vi "Test.vi"() -> ()   [LabVIEW 2017]
doc: "This VI is called when test mode begins, and will automatically be terminated when it ends. You can add manual or automatic tests and invoke them from the dashboard."
uses:
  <vilib>/Rock Robotics/WPI/Utilities/WPI_GetSetVariantRefNum.vi
panel:
  out "Elapsed Time (s) 2":dbl caption="Elapsed Time (s)"
  out "Elapsed Time (s)":dbl
  out "Distance 24":dbl
  out "Distance 23":dbl
  out "Distance 22":dbl
  out "Distance 21":dbl
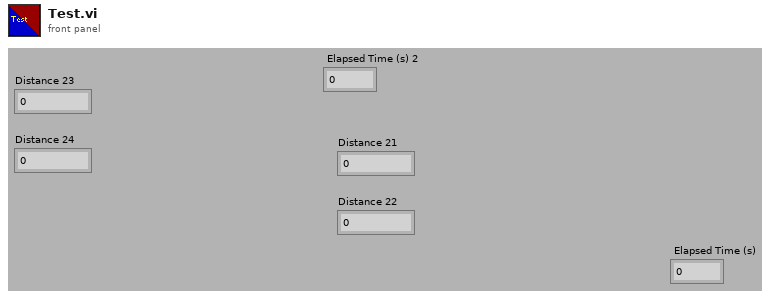
[diagram p1: front panel]
types:
  T1 = typedef "WPI_EncoderDevRef.ctl" = cluster{"DevStatus":errorcluster, "EncoderIndex":T2, "CounterIndex":T3, "DistancePerCount":dbl, "Decoding Type":T4}
  T2 = typedef "FPGA_EncoderIdx.ctl" = enum8{"Enc 0", "Enc 1", "Enc 2", "Enc 3", "Enc 4", "Enc 5", "Enc 6", "Enc 7", "Invalid"}
  T3 = typedef "FPGA_CounterCtrSystemIndex.ctl" = enum8{"Ctr 0", "Ctr 1", "Ctr 2", "Ctr 3", "Ctr 4", "Ctr 5", "Ctr 6", "Ctr 7", "Invalid"}
  T4 = typedef "WPI_EncoderType.ctl" = enum16{"1x", "2x", "4x"}
  T5 = typedef "WPI_RobotDriveDevRef.ctl" = cluster{"DevStatus":errorcluster, "Motors[]":T6[], "Square Inputs":bool, "Max Output":dbl}
  T6 = typedef "WPI_MotorControlDeviceRef.ctl" = cluster{"DeviceStatus":errorcluster, "Type":T7, "PWM":cluster{"PWM Channel":T8, "DeadBand":T9}, "CAN":cluster{"Device Number":u8, "SetOutput VI Ref":variant, "GetOutput VI Ref":variant, "Enable VI Ref":variant, "Disable VI Ref":variant, "Data":variant}, "Invert":bool, "DIO PWM":cluster{"PWM \"Enable\" Channel":T8, "DIOChannel":T10, "PWM Rate":dbl}}
  T7 = typedef "WPI_MotorControlType.ctl" = enum16{"PWM", "CAN", "DIO PWM"}
  T8 = typedef "FPGA_DIOPWMChannel.ctl" = enum8{"PWM 0", "PWM 1", "PWM 2", "PWM 3", "PWM 4", "PWM 5", "PWM 6", "PWM 7", "PWM 8", "PWM 9", "PWM MXP 0", "PWM MXP 1", "PWM MXP 2", "PWM MXP 3", "PWM MXP 4", "PWM MXP 5", "PWM MXP 6", "PWM MXP 7", "PWM MXP 8", "PWM MXP 9", "Invalid"}
  T9 = typedef "WPI_PWMDeadband.ctl" = cluster{"Name":string, "maxPositivePwm":i32, "minPositivePwm":i32, "centerPwm":i32, "maxNegativePwm":i32, "minNegativePwm":i32, "angularRange":u16}
  T10 = typedef "FPGA_DIOChannel.ctl" = enum8{"DIO 0", "DIO 1", "DIO 2", "DIO 3", "DIO 4", "DIO 5", "DIO 6", "DIO 7", "DIO 8", "DIO 9", "DIO MXP 0", "DIO MXP 1", "DIO MXP 2", "DIO MXP 3", "DIO MXP 4", "DIO MXP 5", "DIO MXP 6", "DIO MXP 7", "DIO MXP 8", "DIO MXP 9", "DIO MXP 10", "DIO MXP 11", "DIO MXP 12", "DIO MXP 13", "DIO MXP 14", "DIO MXP 15", "SPI Port CS1", "SPI Port CS2", "SPI Port CS3", "SPI Port MISO", "SPI Port MOSI", "Invalid"}
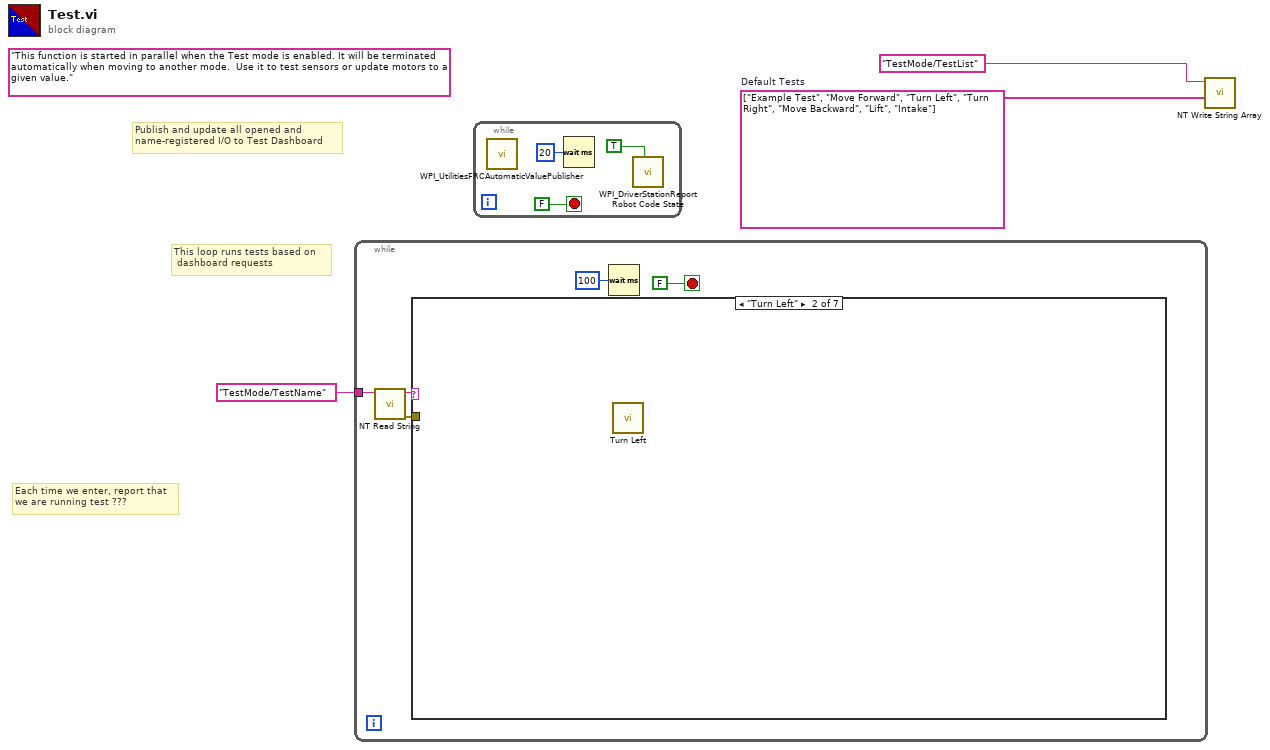
[diagram p0: block diagram]
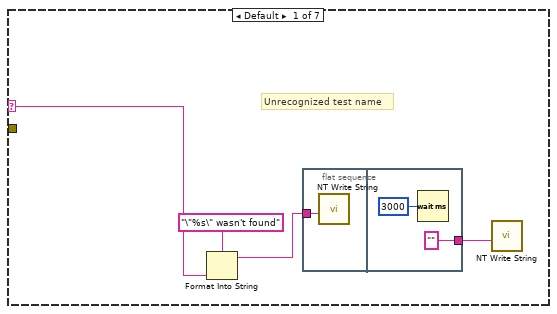
[diagram p2: hidden frame]
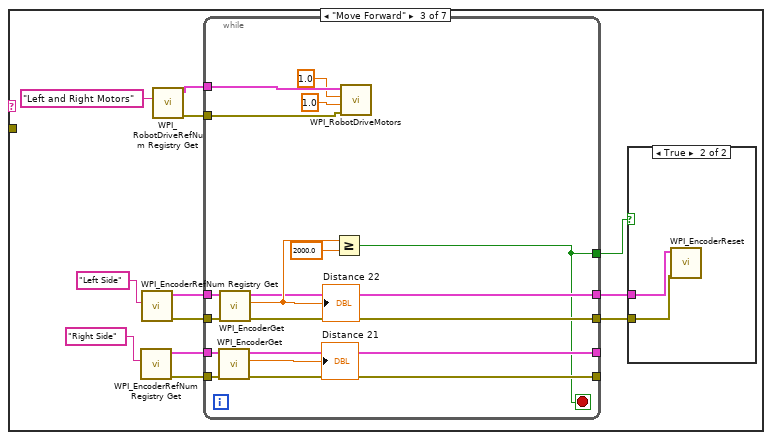
[diagram p3: hidden frame]
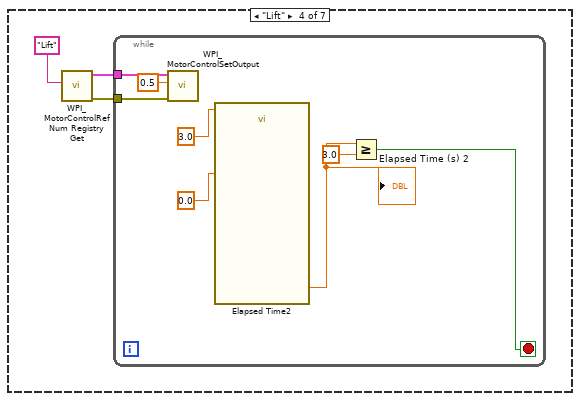
[diagram p5: hidden frame]
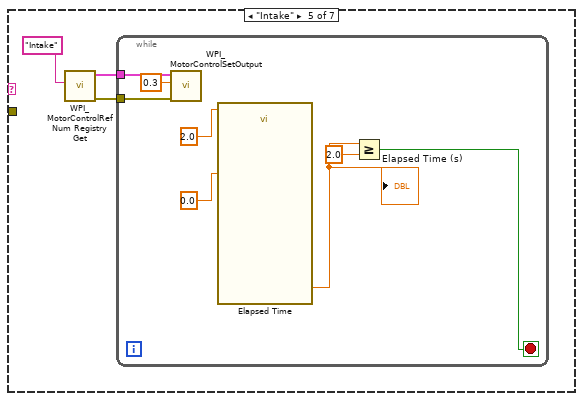
[diagram p6: hidden frame]
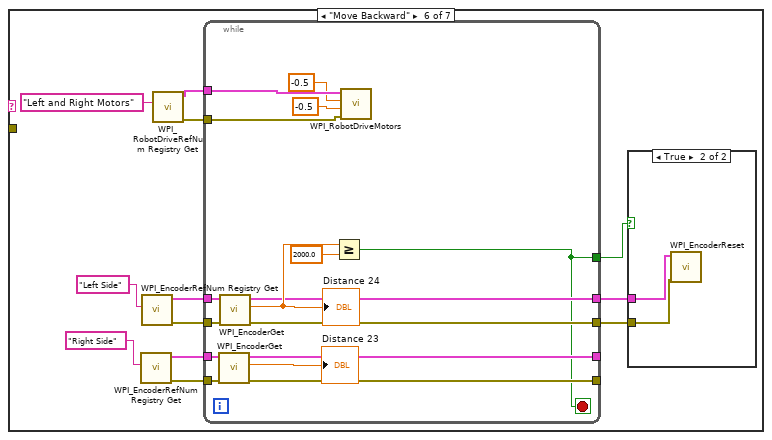
[diagram p7: hidden frame]
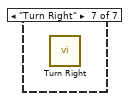
[diagram p9: hidden frame]
diagram:
  w2 = string[] ["Example Test", "Move Forward", "Turn Left", "Turn Right", "Move Backward", "Lift", "Intake"]  # Default Tests
  (unwired) "This function is started in parallel when the Test mode is enabled. It will be terminated automatically when moving to another mode.  Use it to test sensors or update motors to a given value."
  # "This loop runs tests based on \n dashboard requests"
  # "Publish and update all opened and\nname-registered I/O to Test Dashboard"
  # "Each time we enter, report that\nwe are running test ???"
  n1 = while {
    tunnel: "TestMode/TestName" ("Name") -> [w5]
    stop <- FALSE stop-if-true
    n2 = call <vilib>:"NT Read String.vi"("Name"=w5) -> ("error out"=w4:errorcluster, "String"=w6:string)  [unwired: 9 in]
    n3 = case shown="\"Turn Left\"" w6 {
      selector: w6 -> [w12 _ _ _ _ _ _]
      tunnel: w4 -> [_ _ _ _ _ _ _]
      frame Default {
        # "Unrecognized test name"
        n4 = Format Into String(format string="\"%s\" wasn't found" ("Name"), w12) -> (resulting string=w11:string)  [unwired: 2 in, 1 out]
        n5 = flat-sequence {
          tunnel: w11 -> [w13]
          tunnel: ["" ("Name")] -> w9
          frame #0 {
            n6 = call <vilib>:"NT Write String.vi"("String"=w13) -> ()  [unwired: 10 in, 1 out]
          }
          frame #1 {
            n7 = Wait (ms)(milliseconds to wait=u32 3000) -> ()  [unwired: 1 out]
          }
        }
        n8 = call <vilib>:"NT Write String.vi"("String"=w9) -> ()  [unwired: 10 in, 1 out]
      }
      frame "Turn Left" {
        n9 = call "Turn Left.vi"() -> ()  [unwired: 12 in]
      }
      frame "Move Forward" {
        n10 = call <vilib>:"WPI_EncoderRefNum Registry Get.vi"("refnum name"="Right Side") -> ("error out"=w25:errorcluster, "EncoderDevRef"=w24:T1)  [unwired: 9 in]
        n11 = call <vilib>:"WPI_EncoderRefNum Registry Get.vi"("refnum name"="Left Side") -> ("error out"=w26:errorcluster, "EncoderDevRef"=w27:T1)  [unwired: 9 in]
        n12 = call <vilib>:"WPI_RobotDriveRefNum Registry Get.vi"("refnum name"="Left and Right Motors") -> ("error out"=w19:errorcluster, "RobotDriveDevRef"=w20:T5)  [unwired: 9 in]
        n13 = while {
          tunnel: w27 -> [w45]
          tunnel: w26 -> [w44]
          tunnel: w24 -> [w41]
          tunnel: w25 -> [w42]
          tunnel: [w38] -> w22
          tunnel: [w37] -> w21
          tunnel: [w36] -> _
          tunnel: [w35] -> _
          tunnel: [w34] -> w23
          tunnel: w20 -> [w33]
          tunnel: w19 -> [w32]
          stop <- w34 stop-if-true
          n14 = call <vilib>:"WPI_EncoderGet.vi"("error in (no error)"=w42, "EncoderDevRef"=w41) -> ("error out"=w35:errorcluster, "Distance"=→"Distance 21":dbl, "EncoderDevRef"=w36:T1)  [unwired: 4 in, 3 out]
          n15 = call <vilib>:"WPI_EncoderGet.vi"("error in (no error)"=w44, "EncoderDevRef"=w45) -> ("error out"=w37:errorcluster, "Distance"=w40:dbl, "EncoderDevRef"=w38:T1)  [unwired: 4 in, 3 out]
          "Distance 22" <- w40
          n16 = Greater Or Equal?(x=w40, y=2000.0) -> (x >= y?=w34:bool)
          n17 = call <vilib>:"WPI_RobotDriveMotors.vi"("error in (no error)"=w32, "RightSpeed"=1.0, "LeftSpeed"=1.0, "RobotDriveDevRef"=w33) -> ()  [unwired: 5 in, 3 out]
        }
        n18 = case shown="True" w23 {
          tunnel: w22 -> [_ w29]
          tunnel: w21 -> [_ w28]
          frame False {
          }
          frame True {
            n19 = call <vilib>:"WPI_EncoderReset.vi"("error in (no error)"=w28, "EncoderDevRef"=w29) -> ()  [unwired: 8 in, 2 out]
          }
        }
      }
      frame "Lift" {
        n20 = call <vilib>:"WPI_MotorControlRefNum Registry Get.vi"("refnum name"="Lift") -> ("error out"=w47:errorcluster, "MotorControlDevRef"=w48:T6)  [unwired: 9 in]
        n21 = while {
          tunnel: w47 -> [w56]
          tunnel: w48 -> [w55]
          stop <- w49 stop-if-true
          n22 = call <vilib>:"WPI_MotorControlSetOutput.vi"("error in (no error)"=w56, "Output"=0.5, "MotorControlDevRef"=w55) -> ()  [unwired: 6 in, 3 out]
          n23 = call "Elapsed Time2"("Time Target (s)"=3.0, "Set Start Time (s)"=0.0) -> ("Elapsed Time (s)"=w53:dbl)  [unwired: 10 in, 7 out]
          "Elapsed Time (s) 2" <- w53
          n24 = Greater Or Equal?(x=w53, y=3.0) -> (x >= y?=w49:bool)
        }
      }
      frame "Intake" {
        n25 = call <vilib>:"WPI_MotorControlRefNum Registry Get.vi"("refnum name"="Intake") -> ("error out"=w58:errorcluster, "MotorControlDevRef"=w57:T6)  [unwired: 9 in]
        n26 = while {
          tunnel: w58 -> [w67]
          tunnel: w57 -> [w66]
          stop <- w60 stop-if-true
          n27 = call <vilib>:"WPI_MotorControlSetOutput.vi"("error in (no error)"=w67, "Output"=0.3, "MotorControlDevRef"=w66) -> ()  [unwired: 6 in, 3 out]
          n28 = call "Elapsed Time"("Time Target (s)"=2.0, "Set Start Time (s)"=0.0) -> ("Elapsed Time (s)"=w64:dbl)  [unwired: 10 in, 7 out]
          "Elapsed Time (s)" <- w64
          n29 = Greater Or Equal?(x=w64, y=2.0) -> (x >= y?=w60:bool)
        }
      }
      frame "Move Backward" {
        n30 = call <vilib>:"WPI_EncoderRefNum Registry Get.vi"("refnum name"="Right Side") -> ("error out"=w73:errorcluster, "EncoderDevRef"=w74:T1)  [unwired: 9 in]
        n31 = call <vilib>:"WPI_EncoderRefNum Registry Get.vi"("refnum name"="Left Side") -> ("error out"=w72:errorcluster, "EncoderDevRef"=w71:T1)  [unwired: 9 in]
        n32 = call <vilib>:"WPI_RobotDriveRefNum Registry Get.vi"("refnum name"="Left and Right Motors") -> ("error out"=w79:errorcluster, "RobotDriveDevRef"=w78:T5)  [unwired: 9 in]
        n33 = while {
          tunnel: w71 -> [w97]
          tunnel: w72 -> [w96]
          tunnel: w74 -> [w93]
          tunnel: w73 -> [w94]
          tunnel: [w90] -> w76
          tunnel: [w89] -> w77
          tunnel: [w88] -> _
          tunnel: [w87] -> _
          tunnel: [w86] -> w75
          tunnel: w78 -> [w85]
          tunnel: w79 -> [w84]
          stop <- w86 stop-if-true
          n34 = call <vilib>:"WPI_EncoderGet.vi"("error in (no error)"=w94, "EncoderDevRef"=w93) -> ("error out"=w87:errorcluster, "Distance"=→"Distance 23":dbl, "EncoderDevRef"=w88:T1)  [unwired: 4 in, 3 out]
          n35 = call <vilib>:"WPI_EncoderGet.vi"("error in (no error)"=w96, "EncoderDevRef"=w97) -> ("error out"=w89:errorcluster, "Distance"=w92:dbl, "EncoderDevRef"=w90:T1)  [unwired: 4 in, 3 out]
          "Distance 24" <- w92
          n36 = Greater Or Equal?(x=w92, y=2000.0) -> (x >= y?=w86:bool)
          n37 = call <vilib>:"WPI_RobotDriveMotors.vi"("error in (no error)"=w84, "RightSpeed"=-0.5, "LeftSpeed"=-0.5, "RobotDriveDevRef"=w85) -> ()  [unwired: 5 in, 3 out]
        }
        n38 = case shown="True" w75 {
          tunnel: w76 -> [_ w81]
          tunnel: w77 -> [_ w80]
          frame False {
          }
          frame True {
            n39 = call <vilib>:"WPI_EncoderReset.vi"("error in (no error)"=w80, "EncoderDevRef"=w81) -> ()  [unwired: 8 in, 2 out]
          }
        }
      }
      frame "Turn Right" {
        n40 = call "Turn Right.vi"() -> ()  [unwired: 12 in]
      }
    }
    n41 = Wait (ms)(milliseconds to wait=u32 100) -> ()  [unwired: 1 out]
  }
  n42 = while {
    stop <- FALSE stop-if-true
    n43 = call <vilib>:"WPI_UtilitiesFRCAutomaticValuePublisher.vi"() -> ()  [unwired: 12 in]
    n44 = Wait (ms)(milliseconds to wait=u32 20) -> ()  [unwired: 1 out]
    n45 = call <vilib>:"WPI_DriverStationReport Robot Code State.vi"("Test"=TRUE ("Autonomous")) -> ()  [unwired: 10 in, 1 out]
  }
  n46 = call <vilib>:"NT Write String Array.vi"("String Array"=w2, "Name"="TestMode/TestList") -> ()  [unwired: 9 in, 1 out]
